vi "Timing Parameters DAO.vi"(7 "config ref in":T1, 8 "error in (no error)":errorcluster, 10 "Application Timing and Logging In":T3, 11 "Actions":T2) -> (0 "error out":errorcluster, 3 "Application Timing and Logging Out":T3, 6 "config ref out":T1)   [LabVIEW 2013]
uses:
  Timing & Logging Parameters.ctl
  Timing Parameters.ctl
  Metadata/Persistant DAO Actions.ctl
  <vilib>/Utility/config.llb/Config Data RefNum.ctl
  <vilib>/Utility/config.llb/NI_LVConfig.lvlib
panel:
  # "Interval is in Seconds\nRate is in Samples per Second"
  # "Interval is in Seconds\nRate is in Samples per Second"
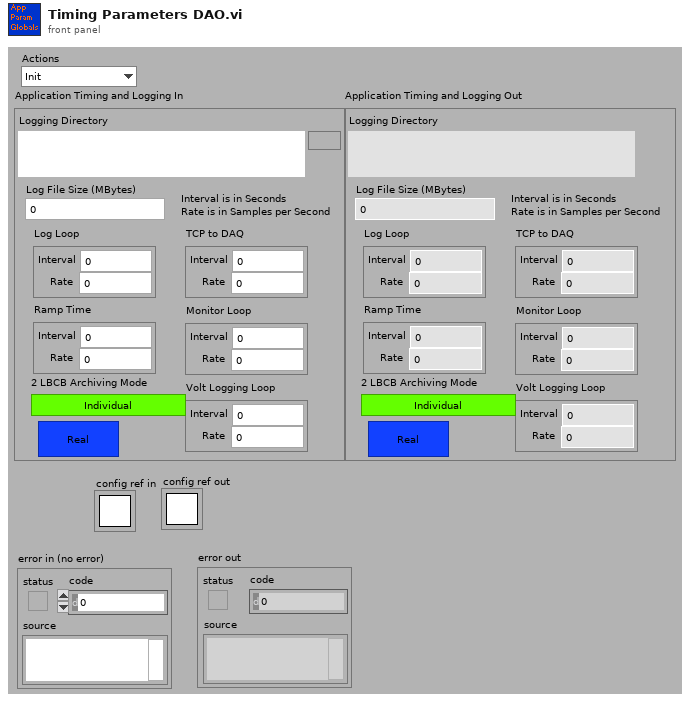
[diagram p1: front panel]
types:
  T1 = typedef "NI_LVConfig.lvlib/Config Data RefNum.ctl" = refnum<k1>
  T2 = typedef "Persistant DAO Actions.ctl" = enum16{"Init", "Get", "Set", "Load", "Save"}
  T3 = typedef "Timing & Logging Parameters.ctl" = cluster{"Monitor Loop":T4, "Ramp Time":T4, "Log Loop":T4, "TCP to DAQ":T4, "Logging Directory":path, "Log File Size (MBytes)":i64, "Volt Logging Loop":T4, "2 LBCB Archiving Mode":bool, "Fake":bool}
  T4 = typedef "Timing Parameters.ctl" = cluster{"Interval":dbl, "Rate ":dbl}
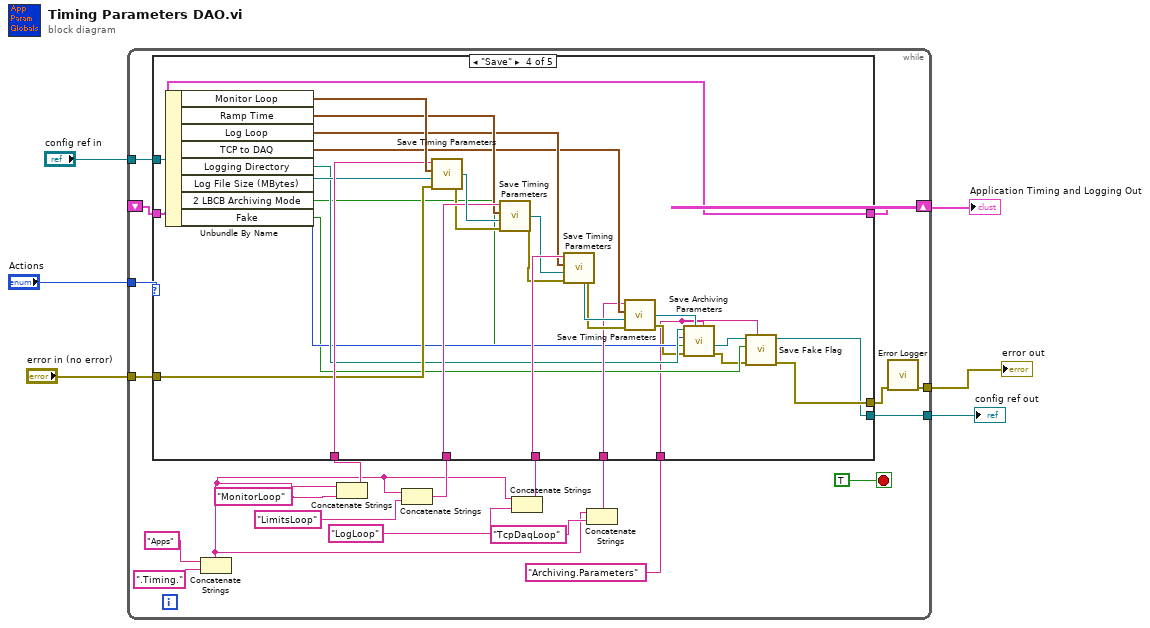
[diagram p0: block diagram]
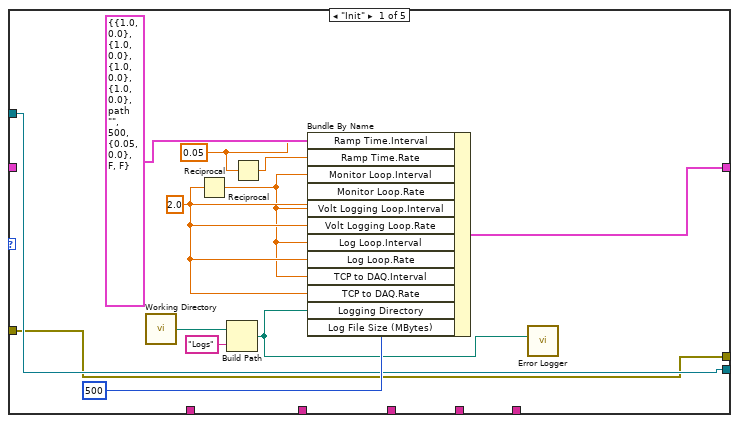
[diagram p2: hidden frame]
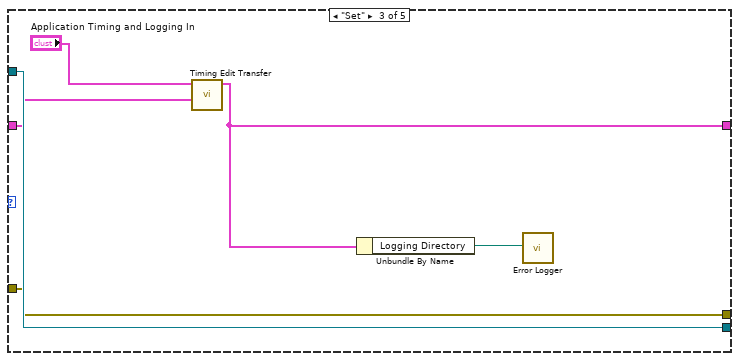
[diagram p4: hidden frame]
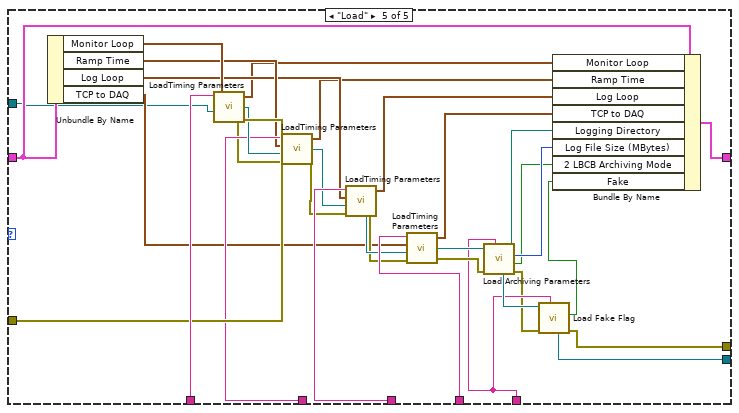
[diagram p5: hidden frame]
diagram:
  n1 = while {
    tunnel: "Actions" -> [w26]
    shift-right: [w25] -> w5
    shift-left: _ -> [w24]
    tunnel: "config ref in" -> [w21]
    tunnel: "error in (no error)" -> [w20]
    tunnel: [w12] -> w2
    tunnel: [w10] -> w1
    stop <- TRUE stop-if-true
    n2 = Concatenate Strings("Apps" ("string"), ".Timing." ("string")) -> (w8:string)
    n3 = Concatenate Strings(w8, "MonitorLoop" ("section")) -> (w22:string)
    n4 = Concatenate Strings(w8, "LimitsLoop" ("section")) -> (w18:string)
    n5 = Concatenate Strings(w8, "LogLoop" ("section")) -> (w15:string)
    n6 = Concatenate Strings(w8, "TcpDaqLoop" ("section")) -> (w14:string)
    n7 = case shown="\"Save\"" w26 {
      tunnel: [w38 w42 w43 w76 w93] -> w25
      tunnel: w24 -> [_ w42 w44 w76 w109]
      tunnel: w22 -> [_ _ _ w74 w107]
      tunnel: w21 -> [w31 w40 w48 w61 w88]
      tunnel: w20 -> [w30 w41 w47 w73 w106]
      tunnel: w18 -> [_ _ _ w71 w104]
      tunnel: w15 -> [_ _ _ w69 w102]
      tunnel: w14 -> [_ _ _ w59 w101]
      tunnel: [w31 w40 w48 w49 w81] -> w12
      tunnel: [w30 w41 w47 w50 w78] -> w11
      tunnel: "Archiving.Parameters" ("string") -> [_ _ _ w51 w80]
      frame "Init" {
        w28 = 0.05 ("Ramp Time.Interval")
        w37 = 2.0 ("Monitor Loop.Sample Rate (Hz)")
        n8 = call "Working Directory.vi"() -> ("Path"=w34:path)  [unwired: 1 out]
        n9 = Reciprocal(x=w37) -> (1/x=w36:dbl)
        n10 = Build Path(base path=w34, name or relative path="Logs") -> (appended path=w32:path)
        n11 = Reciprocal(x=w28) -> (1/x=w29:dbl)
        n12 = Bundle By Name(cluster=T3 {"Monitor Loop"={"Interval"=1.0, "Rate "=0.0}, "Ramp Time"={"Interval"=1.0, "Rate "=0.0}, "Log Loop"={"Interval"=1.0, "Rate "=0.0}, "TCP to DAQ"={"Interval"=1.0, "Rate "=0.0}, "Logging Directory"=path "", "Log File Size (MBytes)"=500, "Volt Logging Loop"={"Interval"=0.05, "Rate "=0.0}, "2 LBCB Archiving Mode"=FALSE, "Fake"=FALSE} ("Application Timing and Logging In"), "Ramp Time.Interval"=w28, "Ramp Time.Rate"=w29, "Monitor Loop.Interval"=w36, "Monitor Loop.Rate"=w37, "Volt Logging Loop.Interval"=w36, "Volt Logging Loop.Rate"=w37, "Log Loop.Interval"=w36, "Log Loop.Rate"=w37, "TCP to DAQ.Interval"=w36, "TCP to DAQ.Rate"=w37, "Logging Directory"=w32, "Log File Size (MBytes)"=i64 500) -> (w38:T3)
        n13 = call "Error Logger.vi"("Logging Directory"=w32) -> ()  [unwired: 1 in, 10 out]
      }
      frame "Get" {
      }
      frame "Set" {
        n14 = call "Timing Edit Transfer.vi"("Application Timing and Logging Old"=w44, "Application Timing and Logging New"="Application Timing and Logging In") -> ("Application Timing and Logging Out"=w43:T3)  [unwired: 9 in]
        n15 = Unbundle By Name(w43) -> ("Logging Directory"=w46:path)
        n16 = call "Error Logger.vi"("Logging Directory"=w46) -> ()  [unwired: 1 in, 10 out]
      }
      frame "Save" {
        n17 = Unbundle By Name(w76) -> ("Monitor Loop"=w75:T4, "Ramp Time"=w70:T4, "Log Loop"=w63:T4, "TCP to DAQ"=w62:T4, "Logging Directory"=w58:path, "Log File Size (MBytes)"=w57:i64, "2 LBCB Archiving Mode"=w56:bool, "Fake"=w54:bool)
        n18 = call "Save Timing Parameters.vi"("error in (no error)"=w73, "refnum"=w61, "Input Cluster"=w75, "section"=w74) -> ("error out"=w66:errorcluster, "refnum out"=w72:T1)  [unwired: 1 out]
        n19 = call "Save Timing Parameters.vi"("error in (no error)"=w66, "refnum"=w72, "Input Cluster"=w70, "section"=w71) -> ("error out"=w65:errorcluster, "refnum out"=w68:T1)  [unwired: 1 out]
        n20 = call "Save Timing Parameters.vi"("error in (no error)"=w65, "refnum"=w68, "Input Cluster"=w63, "section"=w69) -> ("error out"=w64:errorcluster, "refnum out"=w67:T1)  [unwired: 1 out]
        n21 = call "Save Timing Parameters.vi"("error in (no error)"=w64, "refnum"=w67, "Input Cluster"=w62, "section"=w59) -> ("error out"=w55:errorcluster, "refnum out"=w60:T1)  [unwired: 1 out]
        n22 = call "Save Archiving Parameters.vi"("section"=w51, "config ref in"=w60, "error in (no error)"=w55, "2 LBCB Archiving Mode"=w56, "Log File Size (MBytes)"=w57, "Logging Directory"=w58) -> ("error out"=w53:errorcluster, "config ref out"=w52:T1)  [unwired: 4 in]
        n23 = call "Save Fake Flag.vi"("section"=w51, "error in (no error)"=w53, "Fake"=w54, "config ref in"=w52) -> ("error out"=w50:errorcluster, "config ref out"=w49:T1)  [unwired: 5 in]
      }
      frame "Load" {
        n24 = Unbundle By Name(w109) -> ("Monitor Loop"=w108:T4, "Ramp Time"=w103:T4, "Log Loop"=w95:T4, "TCP to DAQ"=w94:T4)
        n25 = call "LoadTiming Parameters.vi"("error in (no error)"=w106, "refnum"=w88, "Input Cluster"=w108, "section"=w107) -> ("error out"=w98:errorcluster, "refnum out"=w105:T1, "Output Cluster"=w92:T4)
        n26 = call "LoadTiming Parameters.vi"("error in (no error)"=w98, "refnum"=w105, "Input Cluster"=w103, "section"=w104) -> ("error out"=w97:errorcluster, "refnum out"=w100:T1, "Output Cluster"=w91:T4)
        n27 = call "LoadTiming Parameters.vi"("error in (no error)"=w97, "refnum"=w100, "Input Cluster"=w95, "section"=w102) -> ("error out"=w96:errorcluster, "refnum out"=w99:T1, "Output Cluster"=w90:T4)
        n28 = call "LoadTiming Parameters.vi"("error in (no error)"=w96, "refnum"=w99, "Input Cluster"=w94, "section"=w101) -> ("error out"=w86:errorcluster, "refnum out"=w87:T1, "Output Cluster"=w89:T4)
        n29 = call "Load Archiving Parameters.vi"("section"=w80, "error in (no error)"=w86, "config ref in"=w87) -> ("error out"=w79:errorcluster, "2 LBCB Archiving Mode"=w83:bool, "Log File Size (MBytes)"=w84:i64, "Logging Directory"=w85:path, "config ref out"=w82:T1)  [unwired: 4 in]
        n30 = call "Load Fake Flag.vi"("section"=w80, "error in (no error)"=w79, "config ref in"=w82) -> ("error out"=w78:errorcluster, "Fake"=w77:bool, "config ref out"=w81:T1)  [unwired: 6 in]
        n31 = Bundle By Name(cluster=w109, "Monitor Loop"=w92, "Ramp Time"=w91, "Log Loop"=w90, "TCP to DAQ"=w89, "Logging Directory"=w85, "Log File Size (MBytes)"=w84, "2 LBCB Archiving Mode"=w83, "Fake"=w77) -> (w93:T3)
      }
    }
    n32 = call "Error Logger.vi"("error in (no error)"=w11) -> ("error out"=w10:errorcluster)  [unwired: 1 in, 9 out]
  }
  "Application Timing and Logging Out" <- w5
  "error out" <- w1
  "config ref out" <- w2
